vi "Enumerate Ports.vi"(9 "Processor":enum16{"SPIKE", "Pi", "Pi_ssh"}(ring), 11 "Python version":string="3.9") -> (0 "error out":errorcluster, 1 "guess":string, 3 "Python":T1, 4 "name":string, 5 "possibilities":string[](array[string]))   [LabVIEW 2021]
uses:
  SerialVIs/PythonCtrl.ctl
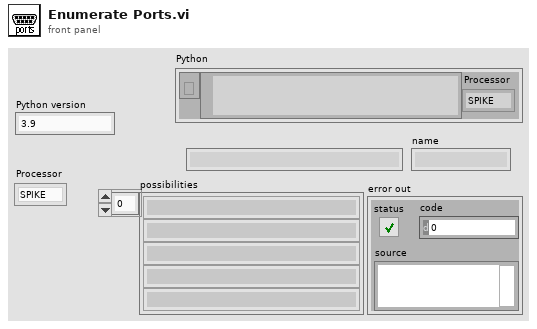
[diagram p1: front panel]
types:
  T1 = typedef "PythonCtrl.ctl" = cluster{"session":refnum<k35>, "PyPath":path, "Processor":enum16{"SPIKE", "Pi", "Pi_ssh"}}
  T2 = cluster{"Refnum out":refnum<k35>, "appended path":path, "Processor":enum16{"SPIKE", "Pi", "Pi_ssh"}}
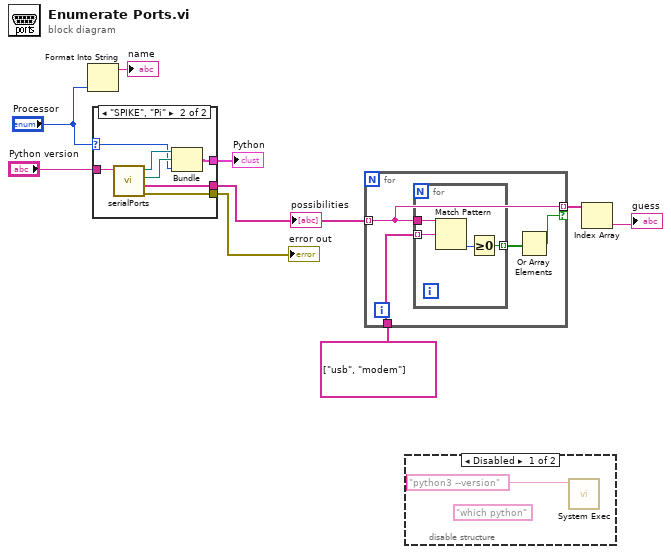
[diagram p0: block diagram]
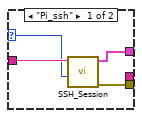
[diagram p2: hidden frame]
diagram:
  n1 = Format Into String("Processor") -> (resulting string=→"name":string)  [unwired: 3 in, 1 out]
  n2 = case shown="\"SPIKE\", \"Pi\"" "Processor" {
    selector: "Processor" -> [w10 w14]
    tunnel: [_ w20] -> w6
    tunnel: [w11 w19] -> w4
    tunnel: "Python version" -> [w13 w18]
    tunnel: [w12 w15] -> w1
    frame "Pi_ssh" {
      n3 = call "SSH_Session.vi"("Processor"=w10, "Python version"=w13) -> ("error out"=w11:errorcluster, "Python"=w12:T1)  [unwired: 8 in]
    }
    frame "SPIKE", "Pi" {
      n4 = call "serialPorts.vi"("Python version"=w18) -> ("error out"=w19:errorcluster, "ports"=w20:string[], "appended path"=w16:path, "Refnum out"=w17:refnum<k35>)  [unwired: 7 in]
      n5 = Bundle("Refnum out"=w17, "appended path"=w16, "Processor"=w14) -> (w15:T2)  [unwired: 1 in]
    }
  }
  "possibilities" <- w6
  "error out" <- w4
  "Python" <- w1
  n6 = for {
    tunnel: w6 -> [w22] mode=indexing
    tunnel: string[] ["usb", "modem"] -> [w24]
    tunnel: [w22] -> w8 mode=indexing if=w21
    n7 = for {
      tunnel: w22 -> [w28]
      tunnel: w24 -> [w27] mode=indexing
      tunnel: [w25] -> w23 mode=indexing
      n8 = Match Pattern(string=w28, regular expression=w27) -> (offset past match=w26:i32)  [unwired: 1 in, 3 out]
      n9 = Greater Or Equal To 0?(x=w26) -> (x >= 0?=w25:bool)
    }
    n10 = Or Array Elements(Boolean array=w23) -> (logical OR=w21:bool)
  }
  n11 = disable-structure shown="Disabled" {
    frame Disabled {
      (unwired) "which python" ("command line")
      n12 = call <vilib>:"System Exec.vi"("command line"="python3 --version") -> ()  [unwired: 7 in, 4 out]
    }
    frame Enabled {
    }
  }
  n13 = Index Array(array=w8) -> (element=→"guess":string)  [unwired: 1 in]
